vi "CRIO write (SubVI).vi"(2 "error IO":errorcluster, 3 "Array":dbl[](array[numeric]), 4 "Port to Write (RT)":enum8{"1", "2", "3", "4"}(ring)=enum."3", 5 "FPGA VI Reference Out 2":refnum<k20>) -> (0 "error out":errorcluster, 1 "FPGA VI Reference Out":refnum<k20>)   [LabVIEW 2011]
uses:
  <vilib>/rvi/errors/niLvFpgaMergeErrorWithErrorCode.vi
  <vilib>/rvi/errors/niLvFpgaAdjustHostInterfaceError.vi
  <vilib>/rvi/interface/nirviReadWriteControl/nirviReadWriteControl.xnode
  FPGA Bitfiles/Mar12misb_FPGATarget_9870InterfaceDMA_04E5410E.lvbitx
  FPGA/9870 Interface DMA (FPGA).vi
  <vilib>/rvi/interface/nirviMethod/nirviMethod.xnode
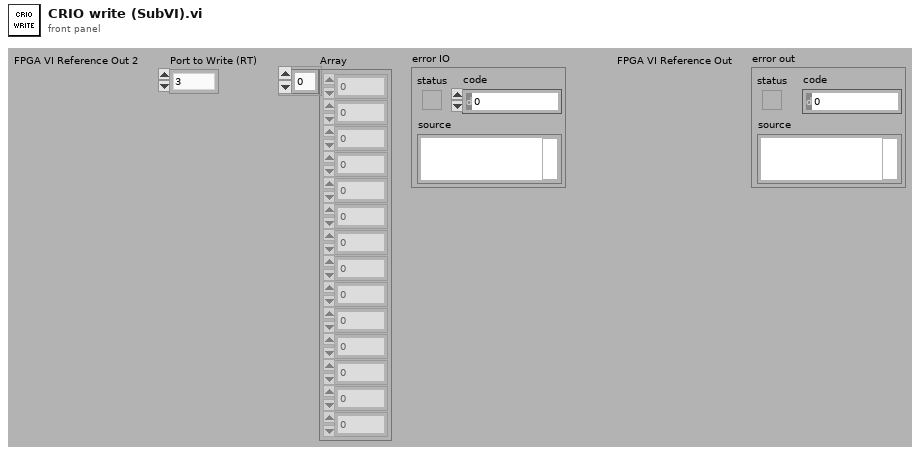
[diagram p1: front panel]
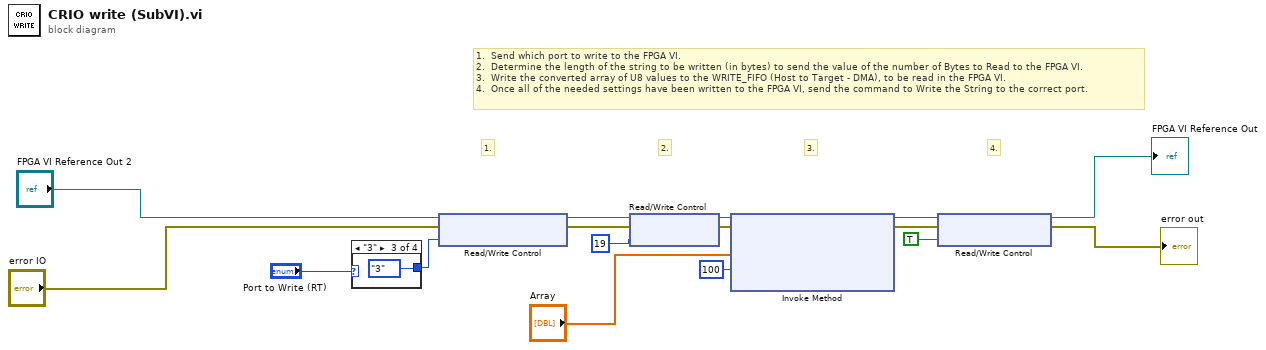
[diagram p0: block diagram]
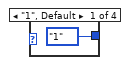
[diagram p2: hidden frame]
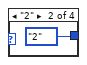
[diagram p3: hidden frame]
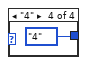
[diagram p4: hidden frame]
diagram:
  # "1.  Send which port to write to the FPGA VI.\n2.  Determine the length of the string to be written (in bytes) to send the value of the number of Bytes to Read to the FPGA VI.\n3.  Write the converted array of U8 values to the WRITE_FIFO (Host to Target - DMA), to be read in the FPGA VI.\n4.  Once all of the needed settings have been written to the FPGA VI, send the command to Write the String to the correct port."
  # "4."
  # "3."
  # "2."
  # "1."
  n1 = case shown="\"3\"" "Port to Write (RT)" {
    tunnel: [enum8{"0", "1", "2", "3", "4"}."1" ("Port To Write (FPGA)") enum8{"0", "1", "2", "3", "4"}."2" ("Port To Write (FPGA)") enum8{"0", "1", "2", "3", "4"}."3" ("Port To Write (FPGA)") enum8{"0", "1", "2", "3", "4"}."4" ("Port To Write (FPGA)")] -> w15
    frame "1", Default {
    }
    frame "2" {
    }
    frame "3" {
    }
    frame "4" {
    }
  }
  n2 = xnode "Read/Write Control"("FPGA VI Reference In"="FPGA VI Reference Out 2", "error in"="error IO", "Port To Write (FPGA)"=w15) -> ("FPGA VI Reference Out"=w11:refnum<k20>, "error out"=w10:errorcluster)
  n3 = xnode "Read/Write Control"("FPGA VI Reference In"=w11, "error in"=w10, "Bytes to Send"=19 ("Timeout (ms)")) -> ("FPGA VI Reference Out"=w13:refnum<k20>, "error out"=w12:errorcluster)
  n4 = xnode "Invoke Method"("FPGA VI Reference In"=w13, "error in"=w12, "Data"="Array", "Timeout (ms)"=100) -> ("FPGA VI Reference Out"=w8:refnum<k20>, "error out"=w9:errorcluster)  [unwired: 1 out]
  n5 = xnode "Read/Write Control"("FPGA VI Reference In"=w8, "error in"=w9, "Write Data (FPGA)"=TRUE) -> ("FPGA VI Reference Out"=→"FPGA VI Reference Out":refnum<k20>, "error out"=→"error out":errorcluster)
